vi "SetArmLimitStatus.vi"(1 "ArmRotateLimit":bool, 2 "ArmExtendLimit":bool) -> ()   [LabVIEW 2017]
uses:
  <vilib>/Rock Robotics/Network Tables/NT Write Boolean.vi
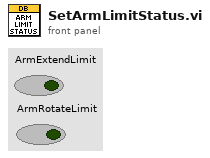
[diagram p1: front panel]
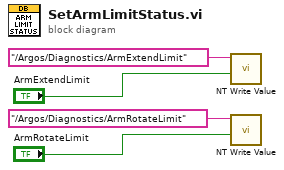
[diagram p0: block diagram]
diagram:
  n1 = call-poly <vilib>:"NT Write Value.vi"("Boolean"="ArmExtendLimit", "Name"="/Argos/Diagnostics/ArmExtendLimit") -> ()  [unwired: 9 in, 1 out]
  n2 = call-poly <vilib>:"NT Write Value.vi"("Boolean"="ArmRotateLimit", "Name"="/Argos/Diagnostics/ArmRotateLimit") -> ()  [unwired: 9 in, 1 out]
